vi "DAQmxBuildTask.vi"(9 "Device port info":T1, 11 "taskNameIn":string) -> (0 "error out":errorcluster)   [LabVIEW 2022 SP3]
uses:
  Device ID port info.ctl
  f383c325-543f-44f0-b992-ec9ac167a994.vi
  <vilib>/DAQmx/create/channels.llb/DAQmx Create Channel (AI-Voltage-Custom with Excitation).vi
  <vilib>/DAQmx/create/channels.llb/DAQmx Create Channel (AI-Voltage-Basic).vi
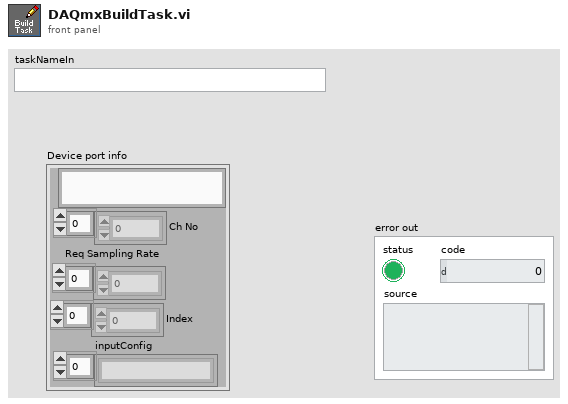
[diagram p1: front panel]
types:
  T1 = typedef "Device ID port info.ctl" = cluster{"Ch No":i16[], "Req Sampling Rate":dbl[], "Port":string, "Index":i32[], "inputConfig":string[]}
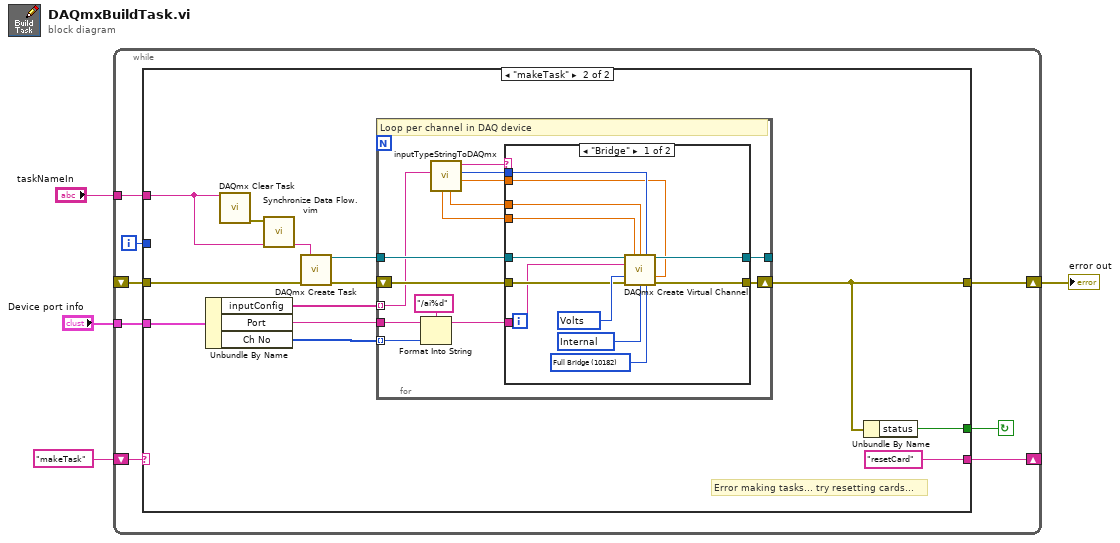
[diagram p0: block diagram]
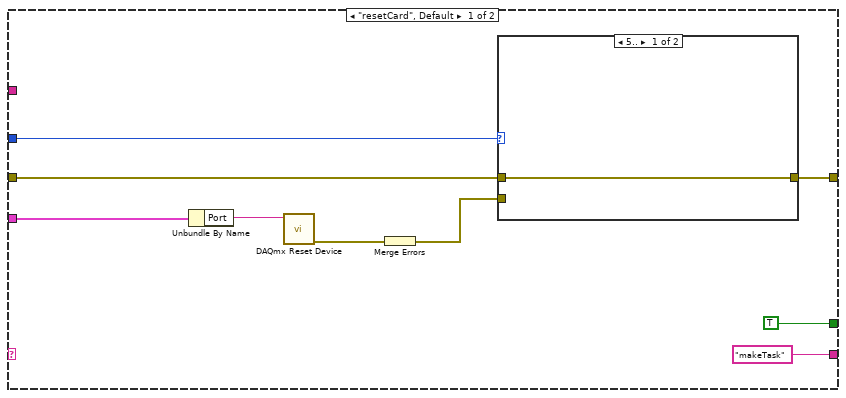
[diagram p2: hidden frame]
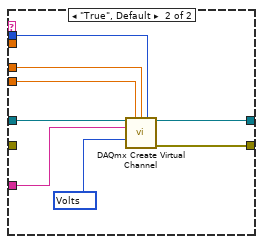
[diagram p4: hidden frame]
diagram:
  n1 = while {
    tunnel: "Device port info" -> [w12]
    shift-right: [w9] -> _
    shift-left: "makeTask" -> [w10]
    shift-right: [w7] -> w3
    shift-left: _ -> [w6]
    tunnel: "taskNameIn" -> [w5]
    i -> [w8]
    stop <- w11 continue-if-true
    n2 = case shown="\"makeTask\"" w10 {
      tunnel: w12 -> [w18 w36]
      tunnel: [TRUE w34] -> w11
      tunnel: ["makeTask" "resetCard"] -> w9
      tunnel: w8 -> [w19 _]
      tunnel: [w15 w33] -> w7
      tunnel: w6 -> [w14 w32]
      tunnel: w5 -> [_ w31]
      frame "resetCard", Default {
        n3 = Unbundle By Name(w18) -> ("Port"=w13:string)
        n4 = call <vilib>:"DAQmx Reset Device.vi"("device in"=w13) -> ("error out"=w17:errorcluster)  [unwired: 14 in]
        n5 = Merge Errors(w17) -> (w16:errorcluster)
        n6 = case shown="5.." w19 {
          tunnel: [w22 w23] -> w15
          tunnel: w16 -> [_ w23]
          tunnel: w14 -> [w22 _]
          frame 5.. {
          }
          frame 0, Default {
          }
        }
      }
      frame "makeTask" {
        # "Error making tasks... try resetting cards..."
        n7 = Unbundle By Name(w36) -> ("inputConfig"=w24:string[], "Port"=w27:string, "Ch No"=w28:i16[])
        n8 = call <vilib>:"DAQmx Clear Task.vi"("task in"=w31) -> ("error out"=w26:errorcluster)  [unwired: 14 in]
        n9 = call "Synchronize Data Flow.vim"("input 4"=w31, "input 1"=w26) -> ("output 4"=w25:string)  [unwired: 2 in, 3 out]
        n10 = call <vilib>:"DAQmx Create Task.vi"("new task name"=w25, "error in"=w32) -> ("task out"=w30:refnum<k21>, "error out"=w29:errorcluster)  [unwired: 3 in, 9 out]
        n11 = for {
          shift-right: [w45] -> w33
          shift-left: w29 -> [w48]
          tunnel: w27 -> [w44]
          tunnel: w28 -> [w43] mode=indexing
          tunnel: w30 -> [w49]
          tunnel: [w46] -> _
          tunnel: w24 -> [w37] mode=indexing
          # "Loop per channel in DAQ device"
          n12 = Format Into String(format string="/ai%d", initial string=w44, w43) -> (resulting string=w47:string)  [unwired: 1 in, 1 out]
          n13 = call "inputTypeStringToDAQmx.vi"("inputConfig"=w37) -> ("Excitation"=w40:dbl, "input terminal configuration"=w42:i32, "inputType"=w41:string, "Span-"=w39:dbl, "Span+"=w38:dbl)  [unwired: 6 in]
          n14 = case shown="\"Bridge\"" w41 {
            tunnel: w49 -> [w62 w67]
            tunnel: w48 -> [w60 _]
            tunnel: w47 -> [w57 w66]
            tunnel: [w56 w69] -> w46
            tunnel: [w55 w68] -> w45
            tunnel: w42 -> [w54 w65]
            tunnel: w40 -> [w53 _]
            tunnel: w38 -> [w52 w64]
            tunnel: w39 -> [w51 w63]
            frame "Bridge" {
              w58 = 10182 items=["Full Bridge"=10182, "Half Bridge"=10187, "Quarter Bridge"=10270, "No Bridge"=10228] ("bridge configuration")
              w59 = 10200 items=["Internal"=10200, "External"=10167, "None"=10230] ("voltage excitation source")
              w61 = 10348 items=["Volts"=10348, "From Custom Scale"=10065] ("units")
              n15 = call-poly <vilib>:"DAQmx Create Virtual Channel.vi"("task in"=w62, "maximum value"=w52, "minimum value"=w51, "input terminal configuration"=w54, "physical channels"=w57, "units"=w61, "voltage excitation value"=w53, "error in"=w60, "voltage excitation source"=w59, "bridge configuration"=w58) -> ("task out"=w56:refnum<k21>, "error out"=w55:errorcluster)  [unwired: 3 in, 1 out]
            }
            frame "True", Default {
              w70 = 10348 items=["Volts"=10348, "From Custom Scale"=10065] ("units")
              n16 = call-poly <vilib>:"DAQmx Create Virtual Channel.vi"("task in"=w67, "maximum value"=w64, "minimum value"=w63, "input terminal configuration"=w65, "physical channels"=w66, "units"=w70) -> ("task out"=w69:refnum<k21>, "error out"=w68:errorcluster)  [unwired: 3 in, 5 out]
            }
          }
        }
        n17 = Unbundle By Name(w33) -> ("status"=w34:bool)
      }
    }
  }
  "error out" <- w3
